vi "故障判别.vi"(5 "TempPointer":u8, 6 "DstPointer":u8, 7 "StdPointer":u8, 8 "SrcPointer":u8) -> (0 "black?":bool, 1 "light?":bool, 2 "flash?":bool, 3 "flickery?":bool, 4 "SumGray":u16)   [LabVIEW 2020]
panel:
  in  "black_size_thres":u32=16
  in  "light_size_thres":u32=16
  in  "flash_size_thres":u32=41472
  in  "flickery_size_thres":u32=165888
  in  "flickery_gray_thres":u8=24
  in  "flash_gray_thres":u8=32
  in  "light_gray_thres":u8=48
  in  "black_gray_thres":u8=40
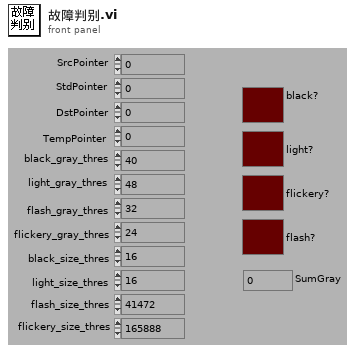
[diagram p1: front panel]
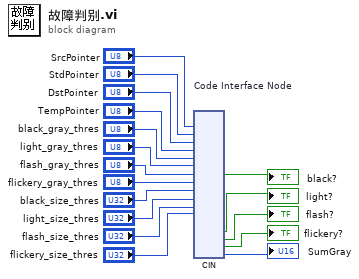
[diagram p0: block diagram]
diagram:
  n1 = cin "Code Interface Node"("SrcPointer", "StdPointer", "DstPointer", "TempPointer", "black_gray_thres", "light_gray_thres", "flash_gray_thres", "flickery_gray_thres", "black_size_thres", "light_size_thres", "flash_size_thres", "flickery_size_thres") -> (→"black?":bool, →"light?":bool, →"flash?":bool, →"flickery?":bool, →"SumGray":u16)  [unwired: 17 in]
